vi "21-1.vi"() -> ()   [LabVIEW 2019, in "21.lvlib"]
uses:
  21.lvlib
  <vilib>/Analysis/1siggen.llb/Ramp Pattern by Delta.vi
  <vilib>/Analysis/NI_AALBase.lvlib
panel:
  in  "Sample?":bool
  out "Loser Score x Rolls":i32
  out "Loser Score":i32
  out "P2 Points":i32
  out "P1 Points":i32
  out "Rolls":i32
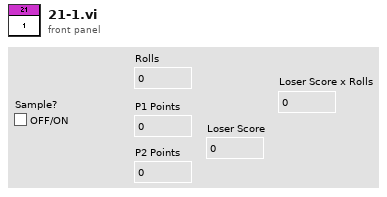
[diagram p1: front panel]
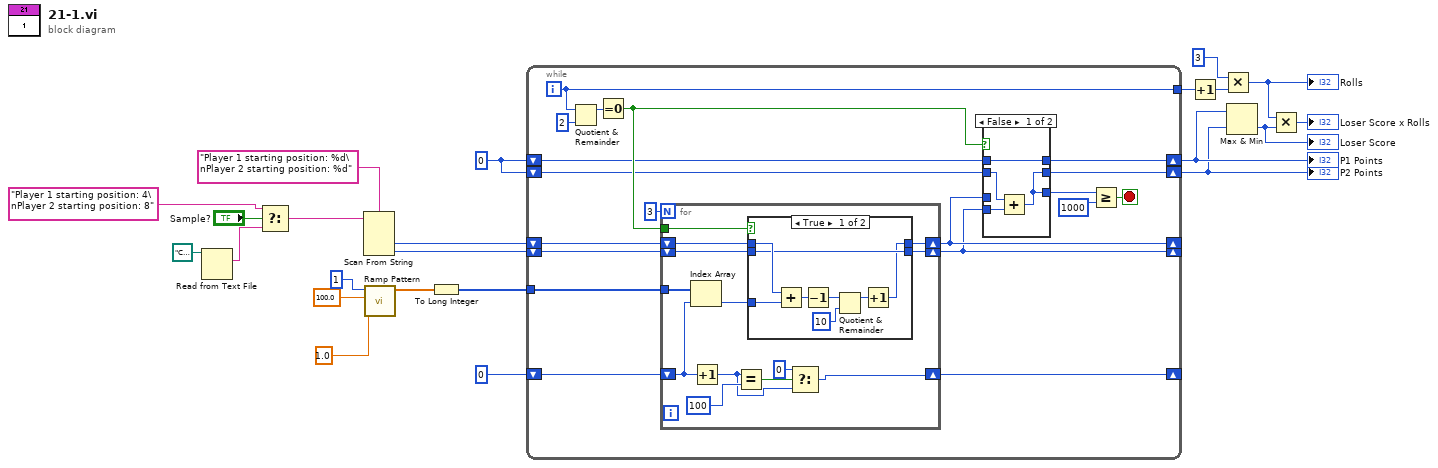
[diagram p0: block diagram]
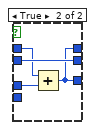
[diagram p2: hidden frame]
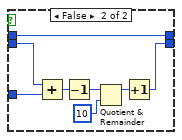
[diagram p3: hidden frame]
diagram:
  w14 = 0
  n1 = Read from Text File(file (use dialog)=path "C:/Users/craig.walker/Documents/GitHub/lv2019-Advent-of-Code-2021/21/input.txt") -> (text=w3:string)  [unwired: 3 in, 3 out]
  n2 = Select(t="Player 1 starting position: 4\nPlayer 2 starting position: 8", s="Sample?", f=w3) -> (s? t:f=w5:string)
  n3 = Scan From String(format string="Player 1 starting position: %d\nPlayer 2 starting position: %d", input string=w5) -> (output 1=w22:i32, output 2=w21:i32)  [unwired: 4 in, 3 out]
  n4 = call-poly <vilib>:"Ramp Pattern.vi"("start"=1.0, "end"=100.0, "delta"=1 ("samples")) -> ("Ramp Pattern"=w20:dbl[])  [unwired: 6 in, 2 out]
  n5 = To Long Integer(number=w20) -> (32bit integer=w16:i32[])
  n6 = while {
    tunnel: w16 -> [w38]
    shift-right: [w41] -> _
    shift-left: 0 -> [w42]
    shift-right: [w29] -> w10
    shift-left: w14 -> [w32]
    shift-right: [w30] -> w9
    shift-left: w14 -> [w31]
    shift-right: [w27] -> _
    shift-left: w21 -> [w39]
    shift-right: [w28] -> _
    shift-left: w22 -> [w40]
    tunnel: [w35] -> w13
    i -> [w35]
    stop <- w24 stop-if-true
    n7 = Quotient & Remainder(x=w35, y=2) -> (x-y*floor(x/y)=w36:i32)  [unwired: 1 out]
    n8 = Equal To 0?(x=w36) -> (x = 0?=w33:bool)
    n9 = for {
      N: 3 -> [_]
      shift-right: [w60] -> w41
      shift-left: w42 -> [w57]
      tunnel: w38 -> [w58]
      tunnel: w33 -> [w51]
      shift-right: [w53] -> w27
      shift-left: w39 -> [w55]
      shift-right: [w52] -> w28
      shift-left: w40 -> [w56]
      n10 = Index Array(array=w58, index=w57) -> (element=w54:i32)
      n11 = Increment(x=w57) -> (x+1=w59:i32)
      n12 = Equal?(x=w59, y=100) -> (x = y?=w62:bool)
      n13 = case shown="True" w51 {
        tunnel: w56 -> [w71 w72]
        tunnel: w55 -> [w69 w74]
        tunnel: w54 -> [w70 w79]
        tunnel: [w69 w73] -> w53
        tunnel: [w64 w72] -> w52
        frame True {
          n14 = Add(x=w71, y=w70) -> (x+y=w66:i32)
          n15 = Decrement(x=w66) -> (x-1=w68:i32)
          n16 = Quotient & Remainder(x=w68, y=10) -> (x-y*floor(x/y)=w65:i32)  [unwired: 1 out]
          n17 = Increment(x=w65) -> (x+1=w64:i32)
        }
        frame False {
          n18 = Add(x=w74, y=w79) -> (x+y=w76:i32)
          n19 = Decrement(x=w76) -> (x-1=w78:i32)
          n20 = Quotient & Remainder(x=w78, y=10) -> (x-y*floor(x/y)=w75:i32)  [unwired: 1 out]
          n21 = Increment(x=w75) -> (x+1=w73:i32)
        }
      }
      n22 = Select(t=0 ("y"), s=w62, f=w59) -> (s? t:f=w60:i32)
    }
    n23 = case shown="False" w33 {
      tunnel: w32 -> [w46 w48]
      tunnel: w31 -> [w45 w50]
      tunnel: [w43 w50] -> w30
      tunnel: [w46 w47] -> w29
      tunnel: w28 -> [_ w49]
      tunnel: w27 -> [w44 _]
      tunnel: [w43 w47] -> w25
      frame False {
        n24 = Add(x=w45, y=w44) -> (x+y=w43:i32)
      }
      frame True {
        n25 = Add(x=w48, y=w49) -> (x+y=w47:i32)
      }
    }
    n26 = Greater Or Equal?(x=w25, y=1000) -> (x >= y?=w24:bool)
  }
  "P1 Points" <- w10
  "P2 Points" <- w9
  n27 = Increment(x=w13) -> (x+1=w12:i32)
  n28 = Multiply(x=3, y=w12) -> (x*y=w7:i32)
  "Rolls" <- w7
  n29 = Max & Min(x=w10, y=w9) -> (min(x,y)=w8:i32)  [unwired: 1 out]
  "Loser Score" <- w8
  n30 = Multiply(x=w7, y=w8) -> (x*y=→"Loser Score x Rolls":i32)
